vi "Test SMPS.vi"() -> ()   [LabVIEW 2015, in "DMA.lvclass"]
uses:
  DMA.lvclass
  DMA.lvclass/DMA.ctl
  <vilib>/Utility/file.llb/Read From Spreadsheet File (DBL).vi
panel:
  out "Waveform Graph":dbl[][](graph)
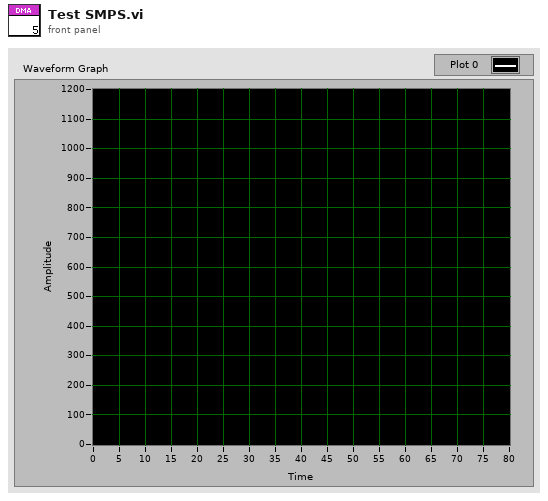
[diagram p1: front panel]
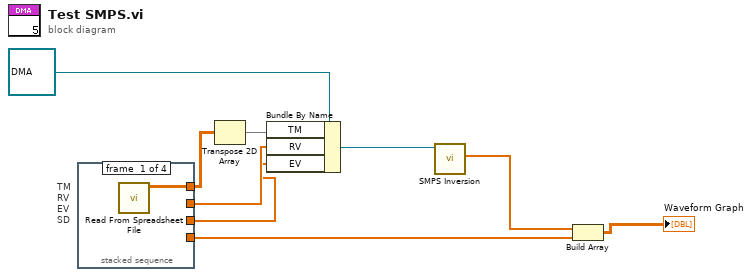
[diagram p0: block diagram]
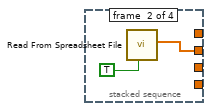
[diagram p2: hidden frame]
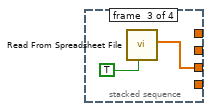
[diagram p3: hidden frame]
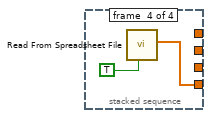
[diagram p4: hidden frame]
diagram:
  # "TM\nRV\nEV\nSD"
  n1 = stacked-sequence {
    tunnel: [w10 _ _ _] -> w5
    tunnel: [_ _ w14 _] -> w7
    tunnel: [_ w12 _ _] -> w8
    tunnel: [_ _ _ w15] -> w2
    frame #0 {
      n2 = call-poly <vilib>:"Read From Spreadsheet File.vi"() -> ("all rows"=w10:dbl[][])  [unwired: 7 in, 4 out]
    }
    frame #1 {
      n3 = call-poly <vilib>:"Read From Spreadsheet File.vi"("transpose (no:F)"=TRUE) -> ("first row"=w12:dbl[])  [unwired: 6 in, 4 out]
    }
    frame #2 {
      n4 = call-poly <vilib>:"Read From Spreadsheet File.vi"("transpose (no:F)"=TRUE) -> ("first row"=w14:dbl[])  [unwired: 6 in, 4 out]
    }
    frame #3 {
      n5 = call-poly <vilib>:"Read From Spreadsheet File.vi"("transpose (no:F)"=TRUE) -> ("first row"=w15:dbl[])  [unwired: 6 in, 4 out]
    }
  }
  n6 = Transpose 2D Array(2D array=w5) -> (transposed array=w4:dbl[][])
  n7 = Bundle By Name(cluster=refnum<class "DMA.lvclass"> refnum ("DMA"), "TM"=w4, "RV"=w8, "EV"=w7) -> (w6:refnum<class "DMA.lvclass">)
  n8 = call "SMPS Inversion.vi"("DMA in"=w6) -> ("IV Out"=w3:sgl[])  [unwired: 8 in, 2 out]
  n9 = Build Array(w3, w2) -> (→"Waveform Graph":dbl[][])
